vi "Thread@TimeCriticalCheck__Parameter.vi"(1 "ParamterIn":string) -> (0 "ParamterOut":string)   [LabVIEW 2020]
panel:
  in  "Confirm":bool
  in  "Message=":string(combo)
  in  "TimeOut":string(combo)
  in  "PortSelect":string(combo)
  # "Thread@TimeCriticalCheck $TimeOut(,$IOLogic,Message=$Message)"
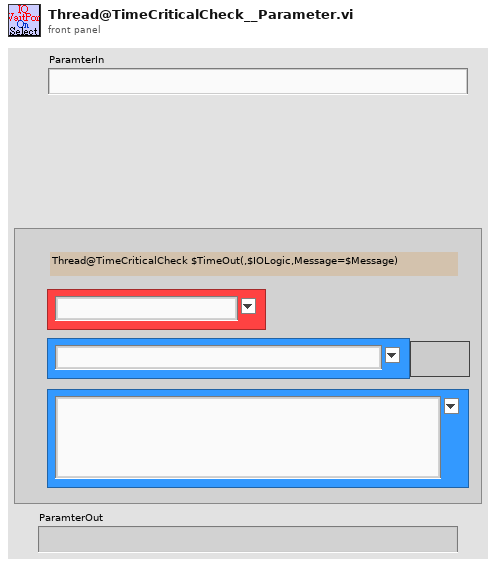
[diagram p1: front panel]
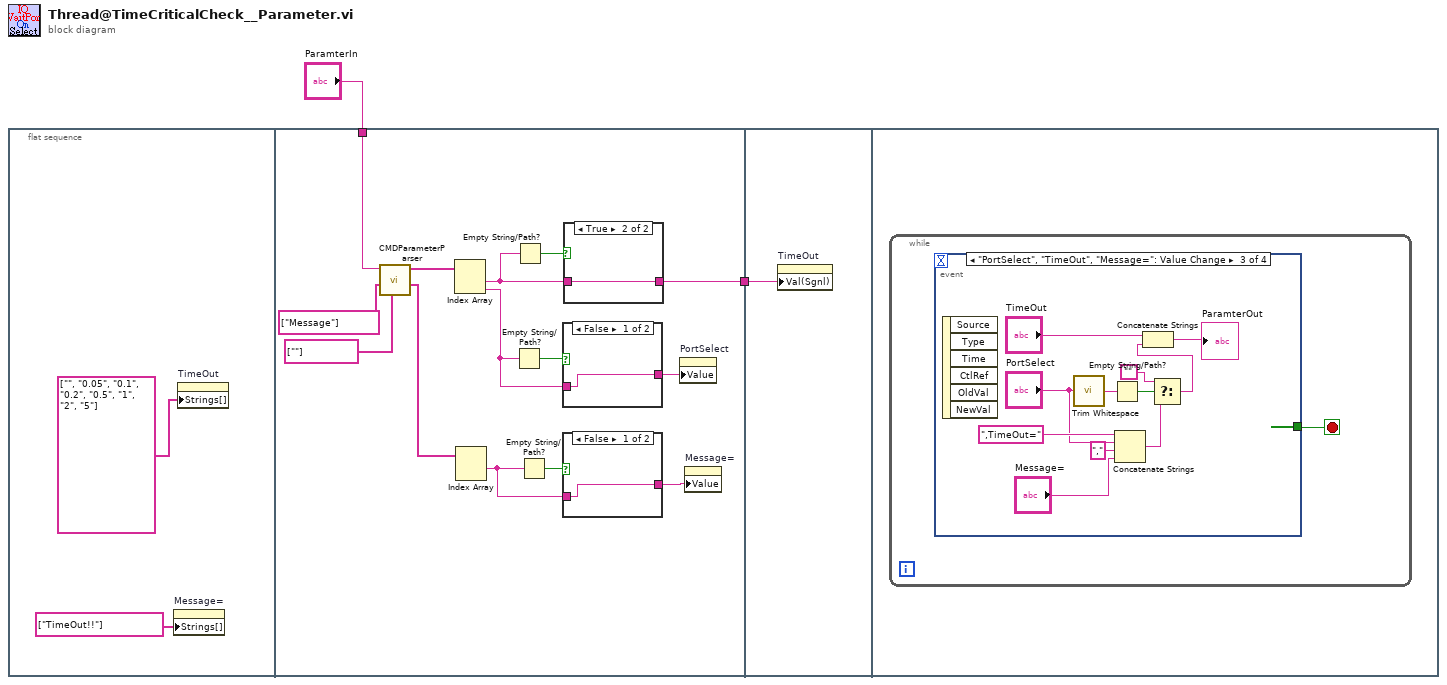
[diagram p0: block diagram]
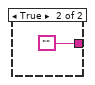
[diagram p2: hidden frame]
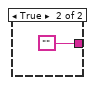
[diagram p3: hidden frame]
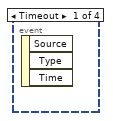
[diagram p5: hidden frame]
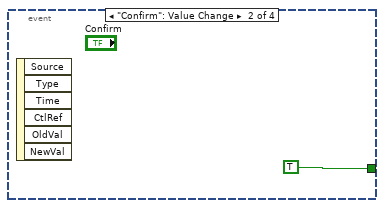
[diagram p6: hidden frame]
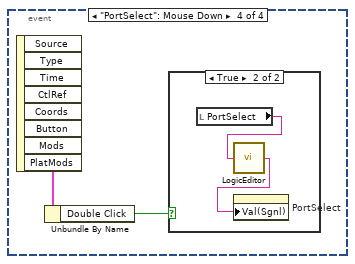
[diagram p7: hidden frame]
diagram:
  n1 = flat-sequence {
    tunnel: "ParamterIn" -> [w11]
    tunnel: [w13] -> w1
    tunnel: w1 -> [w25]
    frame #0 {
      n2 = property on="Message=" class="CmbBox"("Strings[]"=string[] ["TimeOut!!"] ("Strings []")) -> ()  [unwired: 2 in, 2 out]
      n3 = property on="TimeOut" class="CmbBox"("Strings[]"=string[] ["", "0.05", "0.1", "0.2", "0.5", "1", "2", "5"] ("Strings []")) -> ()  [unwired: 2 in, 2 out]
    }
    frame #1 {
      n4 = call "CMDParameterParser.vi"("DeafultValues"=string[] [""], "RequiredKeys"=string[] ["Message"], "CMDParameter"=w11) -> ("KeyValues"=w7:string[], "Input"=w8:string[])  [unwired: 6 in, 1 out]
      n5 = Index Array(array=w8) -> (element #1=w17:string, element #2=w5:string)  [unwired: 2 in]
      n6 = Index Array(array=w7) -> (element #1=w6:string)  [unwired: 2 in, 1 out]
      n7 = Empty String/Path?(string/path=w5) -> (empty?=w16:bool)
      n8 = Empty String/Path?(string/path=w17) -> (empty?=w18:bool)
      n9 = Empty String/Path?(string/path=w6) -> (empty?=w15:bool)
      n10 = case shown="False" w16 {
        tunnel: w5 -> [w21 _]
        tunnel: [w21 ""] -> w12
        frame False {
        }
        frame True {
        }
      }
      n11 = case shown="False" w15 {
        tunnel: w6 -> [w19 _]
        tunnel: [w19 ""] -> w14
        frame False {
        }
        frame True {
        }
      }
      n12 = case shown="True" w18 {
        tunnel: w17 -> [w23 w24]
        tunnel: [w23 w24] -> w13
        frame False {
        }
        frame True {
        }
      }
      n13 = property on="PortSelect" class="CmbBox"("Value"=w12) -> ()  [unwired: 2 in, 2 out]
      n14 = property on="Message=" class="CmbBox"("Value"=w14) -> ()  [unwired: 2 in, 2 out]
    }
    frame #2 {
      n15 = property on="TimeOut" class="CmbBox"("Val(Sgnl)"=w25) -> ()  [unwired: 2 in, 2 out]
    }
    frame #3 {
      n16 = while {
        stop <- w26 stop-if-true
        n17 = event shown="[2] \"PortSelect\", \"TimeOut\", \"Message=\": Value Change" {
          selector: _ -> [_ _ _ _]
          dyn-events: _ -> [_ _ _ _]
          timeout: _ -> [_ _ _ _]
          tunnel: [_ TRUE _ _] -> w26
          event Timeout {
            n18 = event-data() -> ()  [unwired: 1 in, 3 out]
          }
          event "Confirm": Value Change {
            n19 = event-data() -> ()  [unwired: 1 in, 6 out]
          }
          event "PortSelect", "TimeOut", "Message=": Value Change {
            n20 = event-data() -> ()  [unwired: 1 in, 6 out]
            n21 = call <vilib>:"Trim Whitespace.vi"("string"="PortSelect") -> ("trimmed string"=w33:string)  [unwired: 1 in]
            n22 = Empty String/Path?(string/path=w33) -> (empty?=w34:bool)
            n23 = Concatenate Strings(",TimeOut=" ("string"), "PortSelect", "," ("string"), "Message=") -> (w36:string)
            n24 = Select(t="", s=w34, f=w36) -> (s? t:f=w32:string)
            n25 = Concatenate Strings("TimeOut", w32) -> (→"ParamterOut":string)
          }
          event "PortSelect": Mouse Down {
            n26 = event-data() -> ("Mods"=w40:cluster{"Double Click":bool, "Menu Key":bool})  [unwired: 1 in, 7 out]
            n27 = Unbundle By Name(w40) -> ("Double Click"=w39:bool)
            n28 = case shown="True" w39 {
              frame False {
              }
              frame True {
                n29 = local read "PortSelect"() -> (w42:string)
                n30 = call "LogicEditor.vi"("Logic Express"=w42) -> ("LogicExpressOut"=w41:string)
                n31 = property on="PortSelect" class="CmbBox"("Val(Sgnl)"=w41) -> ()  [unwired: 2 in, 2 out]
              }
            }
          }
        }
      }
    }
  }
